vi "Construct.vi"(0 "User Configuration Manager in":refnum<class "User Configuration Manager.lvclass">, 5 "Encryption Type":refnum<class "iEncryption.lvclass">, 11 "error in (no error)":errorcluster) -> (4 "User Configuration Manager out":refnum<class "User Configuration Manager.lvclass">, 15 "error out":errorcluster)   [LabVIEW 2017, in "User Configuration Manager.lvlib" / "User Configuration Manager.lvclass"]
uses:
  User Configuration Manager.lvclass
  iEncryption/iEncryption.lvclass
  <vilib>/gpm_packages/@cs/linked-list/Source/Linked List/Linked List/Linked List.lvclass
  C:/Program Files/National Instruments/LabVIEW 2017/vi.lib/gpm_packages/@cs/linked-list/Source/Linked List/ILinkedList/ILinked List.lvclass
  User Configuration Manager.lvclass/User Configuration Manager.ctl
  Accessors/Write Linked List ID.vi
  Accessors/Write Linked List Ref .vi
  Write Encryption Type.vi
  <vilib>/gpm_packages/@cs/linked-list/Source/Linked List/Linked List Ref/Linked List Ref.lvclass
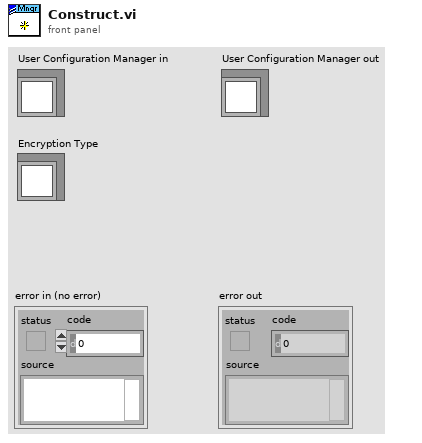
[diagram p1: front panel]
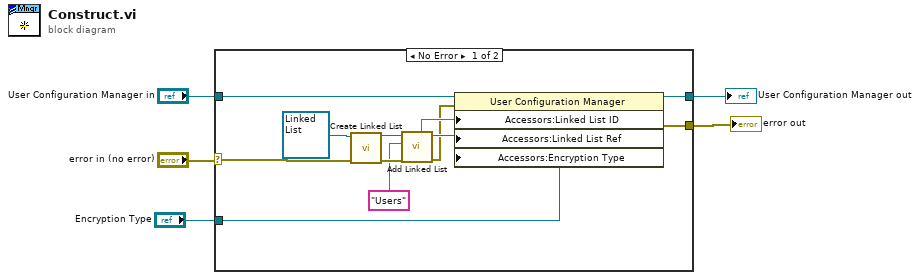
[diagram p0: block diagram]
diagram:
  n1 = case shown="No Error" "error in (no error)" {
    selector: "error in (no error)" -> [w14 w19]
    tunnel: "User Configuration Manager in" -> [w12 w18]
    tunnel: [w11 w18] -> w3
    tunnel: [w7 w19] -> w2
    tunnel: "Encryption Type" -> [w6 _]
    frame No Error {
      n2 = call <vilib>:"Create Linked List.vi"("error in (no error)"=w14, "Linked List"=refnum<class "Linked List.lvclass"> refnum ("Linked Lists.lvlib:Linked List.lvclass")) -> ("error out"=w15:errorcluster, "Linked List Ref"=w17:refnum<data-value>)  [unwired: 8 in]
      n3 = call <vilib>:"Add Linked List.vi"("error in (no error)"=w15, "Name"="Users", "Linked List Ref"=w17) -> ("error out"=w8:errorcluster, "Linked List Ref out"=w9:refnum<data-value>, "Linked List ID out"=w10:string)  [unwired: 5 in, 1 out]
      n4 = property class="User Configuration Manager"(reference=w12, error in=w8, "Accessors:Linked List ID"=w10, "Accessors:Linked List Ref "=w9, "Accessors:Encryption Type"=w6) -> (reference out=w11:refnum<class "User Configuration Manager.lvclass">, error out=w7:errorcluster)
    }
    frame Error {
    }
  }
  "User Configuration Manager out" <- w3
  "error out" <- w2
